vi "Gains.vi"() -> (0 "Rot":T1={"proportional gain (Kc)"=1.0, "integral time (Ti, min)"=0.01, "derivative time (Td, min)"=0.0} {"derivative time (Td, min)" format="%.3f"; "integral time (Ti, min)" format="%.3f"; "proportional gain (Kc)" format="%.3f"}, 3 "Drive":T1={"proportional gain (Kc)"=1.0, "integral time (Ti, min)"=0.01, "derivative time (Td, min)"=0.0} {"derivative time (Td, min)" format="%.3f"; "integral time (Ti, min)" format="%.3f"; "proportional gain (Kc)" format="%.3f"})   [LabVIEW 2014]
uses:
  <vilib>/Rock Robotics/Network Tables/SD Read Numeric Array.vi
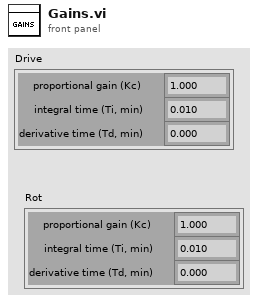
[diagram p1: front panel]
types:
  T1 = cluster{"proportional gain (Kc)":dbl, "integral time (Ti, min)":dbl, "derivative time (Td, min)":dbl}
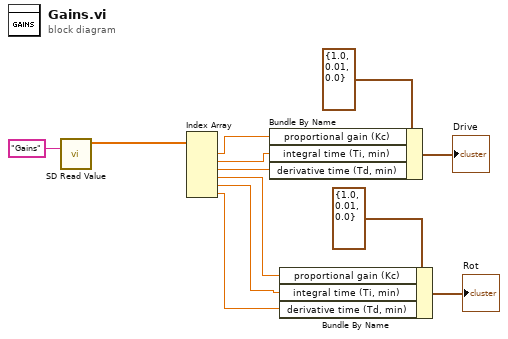
[diagram p0: block diagram]
diagram:
  n1 = call-poly <vilib>:"SD Read Value.vi"("Name"="Gains") -> ("Numeric Array"=w11:dbl[])  [unwired: 8 in, 2 out]
  n2 = Index Array(array=w11) -> (element #1=w10:dbl, element #2=w9:dbl, element #3=w8:dbl, element #4=w3:dbl, element #5=w2:dbl, element #6=w1:dbl)  [unwired: 6 in]
  n3 = Bundle By Name(cluster=T1 {"proportional gain (Kc)"=1.0, "integral time (Ti, min)"=0.01, "derivative time (Td, min)"=0.0} ("PID gains"), "proportional gain (Kc)"=w10, "integral time (Ti, min)"=w9, "derivative time (Td, min)"=w8) -> (→"Drive":T1)
  n4 = Bundle By Name(cluster=T1 {"proportional gain (Kc)"=1.0, "integral time (Ti, min)"=0.01, "derivative time (Td, min)"=0.0} ("PID gains"), "proportional gain (Kc)"=w3, "integral time (Ti, min)"=w2, "derivative time (Td, min)"=w1) -> (→"Rot":T1)
